vi "EMGstats(subvi).vi"(0 "EMG signál":waveform(dbl)) -> (1 "Signál s vlastnostmi":waveform(dbl)[](array[waveform]), 3 "Efektivní hodnota":dbl format="%0.2f")   [LabVIEW 2026]
uses:
  <vilib>/Analysis/3filter.llb/Filter Passband Type.ctl
  <vilib>/Analysis/5stat.llb/RMS (DBL).vi
  <vilib>/Analysis/3filter.llb/Butterworth Filter (DBL).vi
  <vilib>/Analysis/NI_AALBase.lvlib
  <vilib>/ptbypt/NI_PtbyPt.lvlib
  <vilib>/Analysis/NI_AALPro.lvlib
panel:
  out "Celková energie":dbl format="%#_4g"
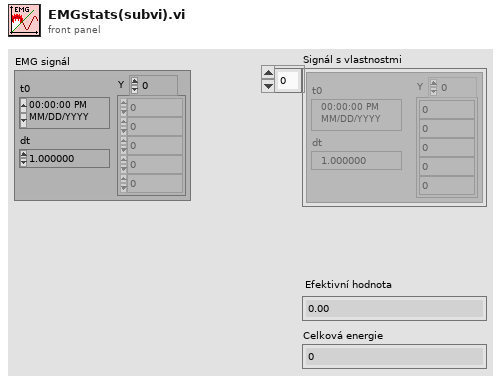
[diagram p1: front panel]
types:
  T1 = typedef "NI_AALBase.lvlib/Filter Passband Type.ctl" = enum32{"Lowpass", "Highpass", "Bandpass", "Bandstop"}
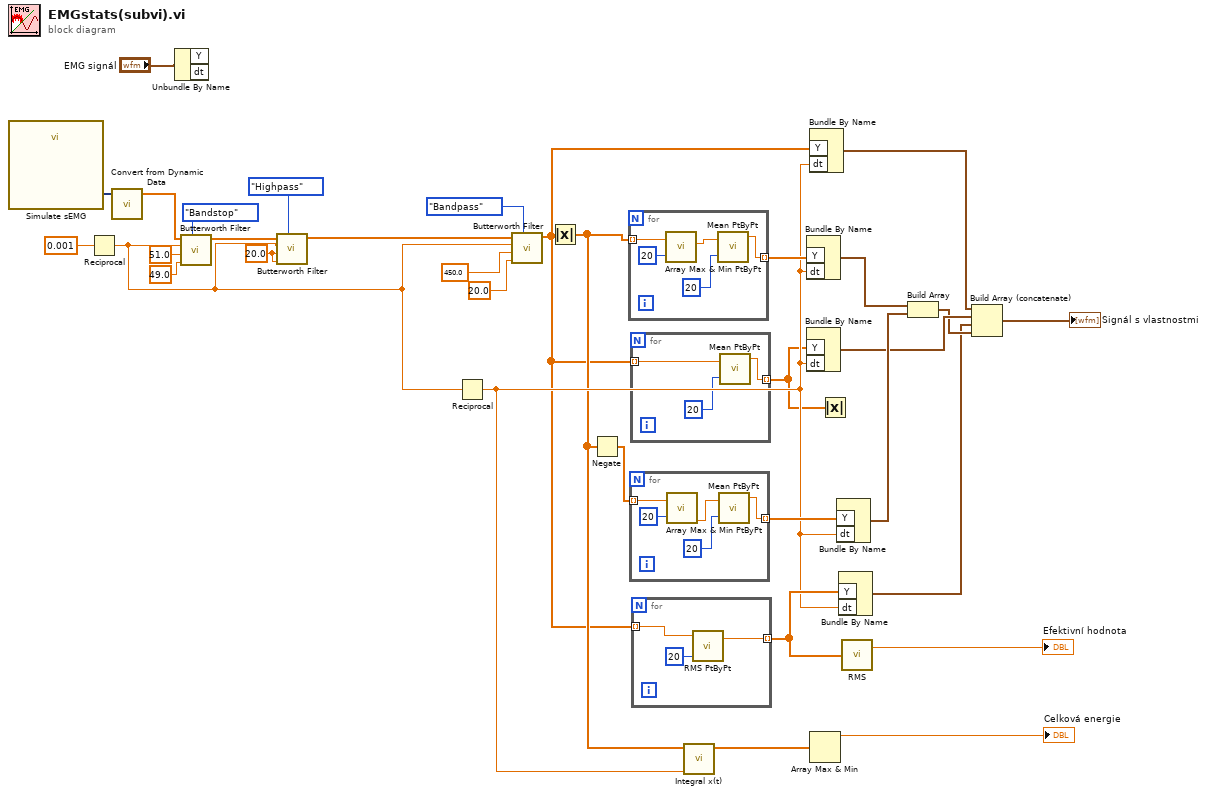
[diagram p0: block diagram]
diagram:
  w5 = 20.0 ("high cutoff freq: fh")
  n1 = call "Simulate sEMG"() -> ("EMG"=w12:dynamicdata)  [unwired: 10 in, 1 out]
  n2 = Reciprocal(x=0.001) -> (1/x=w6:dbl)
  n3 = call "Convert from Dynamic Data"("Dynamic Data Type"=w12) -> ("Array"=w11:dbl[])  [unwired: 3 in]
  n4 = Unbundle By Name("EMG signál") -> ()  [unwired: 2 out]
  n5 = call-poly <vilib>:"Butterworth Filter.vi"("filter type"=Filter_Passband_Type."Bandstop", "low cutoff freq: fl"=49.0, "high cutoff freq: fh"=51.0, "sampling freq: fs"=w6, "X"=w11) -> ("Filtered X"=w7:dbl[])  [unwired: 3 in, 1 out]
  n6 = call-poly <vilib>:"Butterworth Filter.vi"("filter type"=Filter_Passband_Type."Highpass", "low cutoff freq: fl"=w5, "high cutoff freq: fh"=w5, "sampling freq: fs"=w6, "X"=w7) -> ("Filtered X"=w3:dbl[])  [unwired: 3 in, 1 out]
  n7 = Reciprocal(x=w6) -> (1/x=w20:dbl)
  n8 = call-poly <vilib>:"Butterworth Filter.vi"("filter type"=Filter_Passband_Type."Bandpass", "low cutoff freq: fl"=20.0, "high cutoff freq: fh"=450.0, "sampling freq: fs"=w6, "X"=w3) -> ("Filtered X"=w16:dbl[])  [unwired: 3 in, 1 out]
  n9 = Absolute Value(x=w16) -> (abs(x)=w17:dbl[])
  n10 = Negate(x=w17) -> (-x=w27:dbl[])
  n11 = for {
    tunnel: w17 -> [w38] mode=indexing
    tunnel: [w34] -> w30 mode=indexing
    n12 = call <vilib>:"Array Max & Min PtByPt.vi"("input data point"=w38, "sample length"=20) -> ("max value"=w36:dbl)  [unwired: 1 in, 4 out]
    n13 = call <vilib>:"Mean PtByPt.vi"("x"=w36, "sample length"=20) -> ("mean"=w34:dbl)  [unwired: 2 in, 1 out]
  }
  n14 = for {
    tunnel: w27 -> [w43] mode=indexing
    tunnel: [w40] -> w28 mode=indexing
    n15 = call <vilib>:"Array Max & Min PtByPt.vi"("input data point"=w43, "sample length"=20) -> ("min value"=w39:dbl)  [unwired: 1 in, 4 out]
    n16 = call <vilib>:"Mean PtByPt.vi"("x"=w39, "sample length"=20) -> ("mean"=w40:dbl)  [unwired: 2 in, 1 out]
  }
  n17 = for {
    tunnel: w16 -> [w44] mode=indexing
    tunnel: [w45] -> w14 mode=indexing
    n18 = call <vilib>:"Mean PtByPt.vi"("x"=w44, "sample length"=20) -> ("mean"=w45:dbl)  [unwired: 2 in, 1 out]
  }
  n19 = for {
    tunnel: w16 -> [w49] mode=indexing
    tunnel: [w47] -> w23 mode=indexing
    n20 = call <vilib>:"RMS PtByPt.vi"("sample length"=20, "x"=w49) -> ("rms value"=w47:dbl)  [unwired: 2 in, 1 out]
  }
  n21 = call <vilib>:"Integral x(t).vi"("dt"=w20, "X"=w17) -> ("Integral X"=w19:dbl[])  [unwired: 8 in, 1 out]
  n22 = Bundle By Name("Y"=w30, "dt"=w20) -> (w29:waveform(dbl))  [unwired: 1 in]
  n23 = Bundle By Name("Y"=w14, "dt"=w20) -> (w25:waveform(dbl))  [unwired: 1 in]
  n24 = Bundle By Name("Y"=w16, "dt"=w20) -> (w24:waveform(dbl))  [unwired: 1 in]
  n25 = Array Max & Min(array=w19) -> (max value=→"Celková energie":dbl)  [unwired: 3 out]
  n26 = Absolute Value(x=w14) -> ()  [unwired: 1 out]
  n27 = Bundle By Name("Y"=w28, "dt"=w20) -> (w26:waveform(dbl))  [unwired: 1 in]
  n28 = Bundle By Name("Y"=w23, "dt"=w20) -> (w1:waveform(dbl))  [unwired: 1 in]
  n29 = call-poly <vilib>:"RMS.vi"("X"=w23) -> ("rms value"=→"Efektivní hodnota":dbl)  [unwired: 1 out]
  n30 = Build Array(w29, w26) -> (w2:waveform(dbl)[])
  n31 = Build Array (concatenate)(w24, w25, w1, w2) -> (→"Signál s vlastnostmi":waveform(dbl)[])
